vi "LeCroy.Recall Histo Config.vi"(8 "Error In":errorcluster, 10 "Filename (panel.lss)":string="spd-ap-setup-100khz--00000.lss", 11 "LeCroy.Session in":T1) -> (0 "Error Out":errorcluster, 3 "LeCroy.Session out":T1)   [LabVIEW 2018]
uses:
  typedefs/LeCroy.Session.ctl
  Driver/lecroy_wave_series/LeCroy Wave Series/LeCroy Wave Series.lvlib
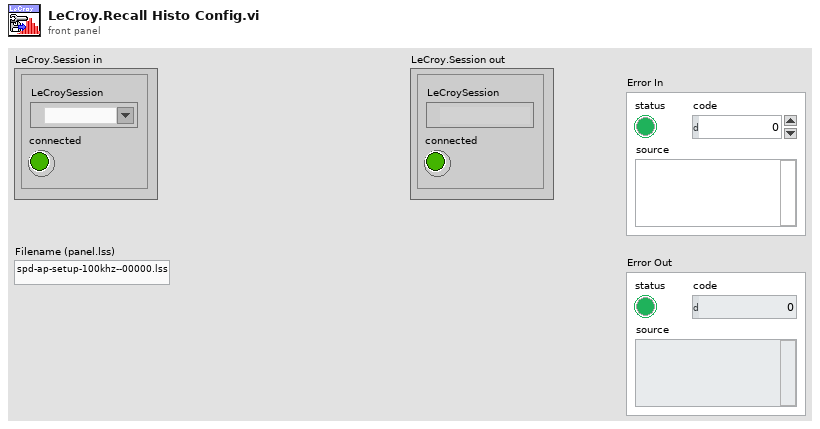
[diagram p1: front panel]
types:
  T1 = typedef "LeCroy.Session.ctl" = cluster{"LeCroySession":refnum<visa-resource-name>, "connected":bool}
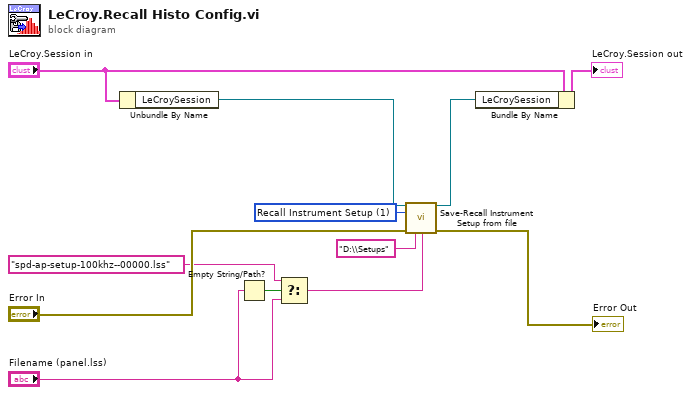
[diagram p0: block diagram]
diagram:
  w10 = u16 1 items=["Save Instrument Setup", "Recall Instrument Setup"] ("Action (0:Save Instrument Setup)")
  n1 = Unbundle By Name("LeCroy.Session in") -> ("LeCroySession"=w8:refnum<visa-resource-name>)
  n2 = Empty String/Path?(string/path="Filename (panel.lss)") -> (empty?=w6:bool)
  n3 = Select(t="spd-ap-setup-100khz--00000.lss" ("Filename (panel.lss)"), s=w6, f="Filename (panel.lss)") -> (s? t:f=w4:string)
  n4 = call "Save-Recall Instrument Setup from file.vi"("VISA resource name"=w8, "Action (0:Save Instrument Setup)"=w10, "error in (no error)"="Error In", "Path (D:\\Setups)"="D:\\Setups" ("Path (D:\\Setups)"), "Filename (panel.lss)"=w4) -> ("VISA resource name out"=w2:refnum<visa-resource-name>, "error out"=→"Error Out":errorcluster)  [unwired: 9 in]
  n5 = Bundle By Name(cluster="LeCroy.Session in", "LeCroySession"=w2) -> (→"LeCroy.Session out":T1)
